vi "Listen.vi"(8 "error in (no error)":errorcluster, 11 "COGNEX IP:Port(recv)":string="192.168.0.30:4001") -> (0 "error out":errorcluster, 1 "f":string, 2 "狀態":string, 3 "Raw data":string, 4 "current time":timestamp, 5 "指示燈":bool)   [LabVIEW 2019, in "Kolmogan Library 1.lvlib"]
uses:
  Kolmogan Library 1.lvlib
  <vilib>/regexp/Match Regular Expression.xnode
panel:
  out "x-y":dbl
  out "length":i32
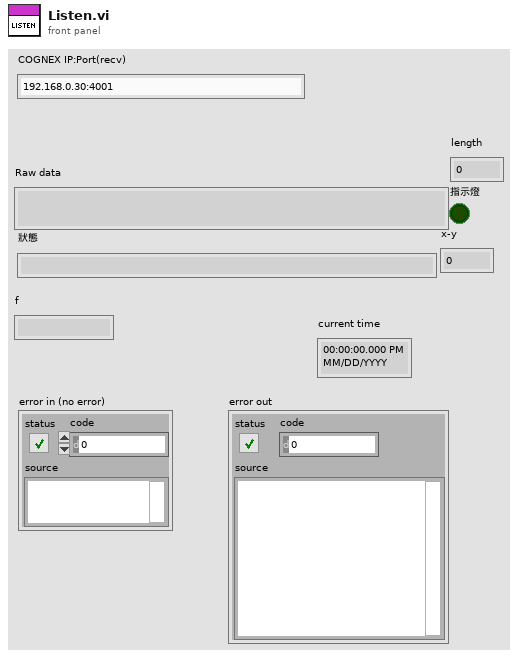
[diagram p1: front panel]
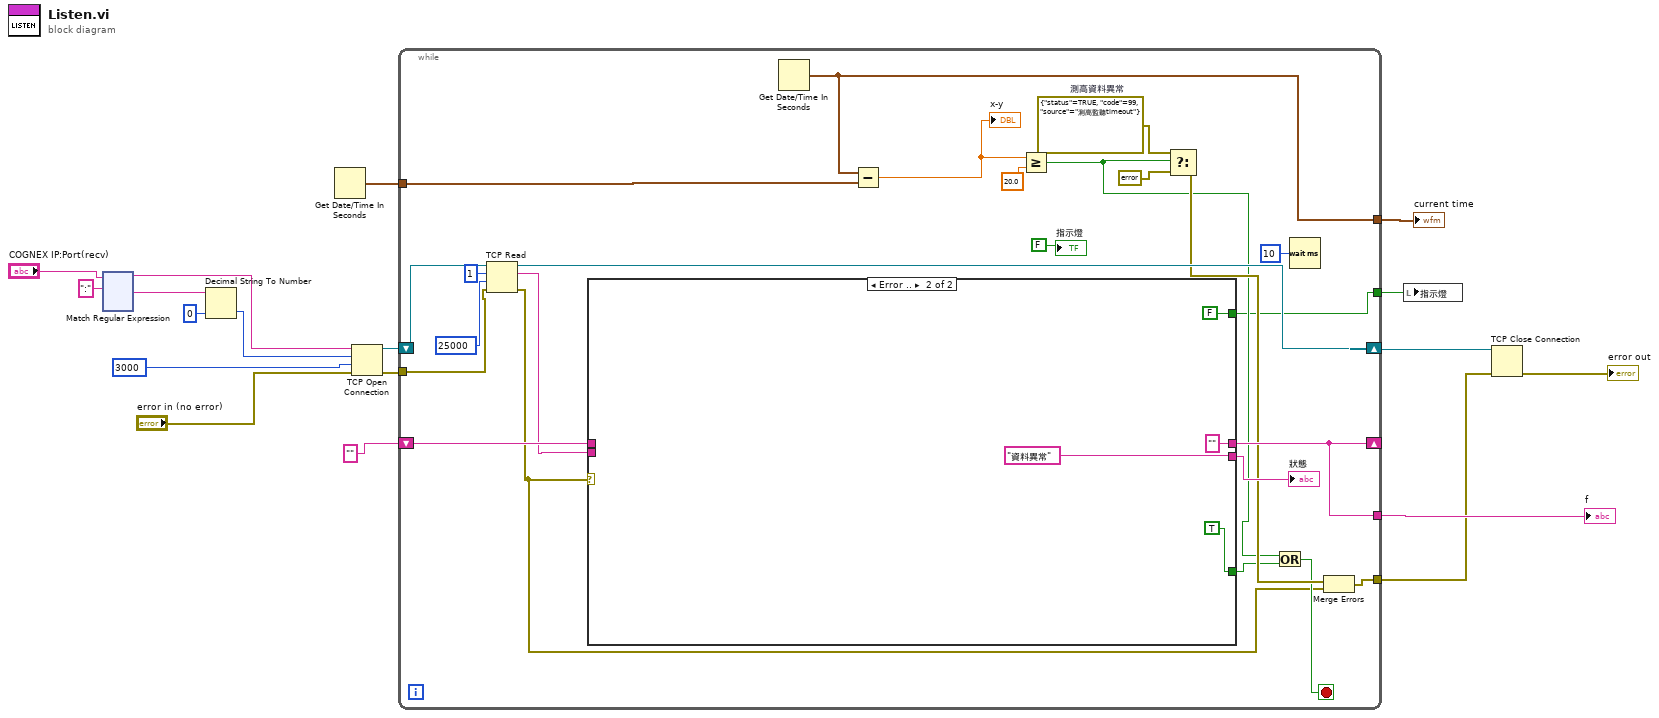
[diagram p0: block diagram]
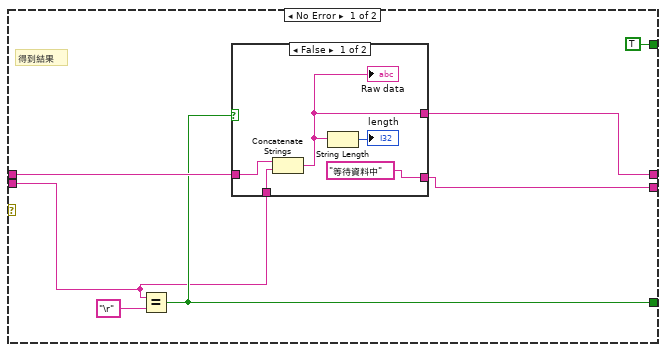
[diagram p2: hidden frame]
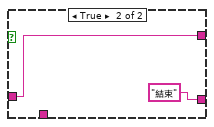
[diagram p3: hidden frame]
diagram:
  n1 = xnode "Match Regular Expression"("input string"="COGNEX IP:Port(recv)", "regular expression"=":") -> ("before match"=w3:string, "after match"=w6:string)  [unwired: 4 in, 3 out]
  n2 = Decimal String To Number(string=w6, default (0L)=u16 0 ("default (0 I32)")) -> (number=w2:u16)  [unwired: 1 in, 1 out]
  n3 = Get Date/Time In Seconds() -> (seconds since 1Jan1904=w8:timestamp)
  n4 = TCP Open Connection(address=w3, remote port or service name=w2, timeout ms (60000)=3000, error in (no error)="error in (no error)") -> (connection ID=w11:refnum<k5>, error out=w13:errorcluster)  [unwired: 1 in]
  n5 = while {
    shift-right: [w38] -> w15
    shift-left: w11 -> [w42]
    shift-right: [w32] -> _
    shift-left: "" ("string") -> [w39]
    tunnel: w13 -> [w37]
    tunnel: [w27] -> w16
    tunnel: [w32] -> w18
    tunnel: [w22] -> w10
    tunnel: [w20] -> w9
    tunnel: w8 -> [w21]
    stop <- w24 stop-if-true
    w28 = errorcluster {"status"=TRUE, "code"=99, "source"="測高監聽timeout"}  # 測高資料異常
    n6 = TCP Read(connection ID=w42, bytes to read=1, error in (no error)=w37, 9:25000 ("timeout ms (25000)")) -> (connection ID out=w38:refnum<k5>, data out=w35:string, error out=w19:errorcluster)  [unwired: 1 in]
    n7 = case shown="Error .." w19 {
      tunnel: w35 -> [w45 _]
      tunnel: w39 -> [w49 _]
      tunnel: [w48 ""] -> w32
      tunnel: [w44 "資料異常" ("f")] -> w33
      tunnel: [w46 TRUE] -> w25
      tunnel: [TRUE ("指示燈") FALSE ("指示燈")] -> w20
      frame No Error {
        # "得到結果"
        n8 = Equal?(x=w45, y="\r") -> (x = y?=w46:bool)
        n9 = case shown="False" w46 {
          tunnel: w49 -> [w54 w56]
          tunnel: [w53 w56] -> w48
          tunnel: w45 -> [w51 _]
          tunnel: ["等待資料中" ("f") "結束" ("t")] -> w44
          frame False {
            n10 = Concatenate Strings(w54, w51) -> (w53:string)
            "Raw data" <- w53
            n11 = String Length(string=w53) -> (length=→"length":i32)
          }
          frame True {
          }
        }
      }
      frame Error {
      }
    }
    "狀態" <- w33
    n12 = Get Date/Time In Seconds() -> (seconds since 1Jan1904=w22:timestamp)
    n13 = Subtract(x=w22, y=w21) -> (x-y=w31:dbl)
    "x-y" <- w31
    n14 = Greater Or Equal?(x=w31, y=20.0) -> (x >= y?=w23:bool)
    n15 = Select(t=w28, s=w23, f=errorcluster {"status"=FALSE, "code"=0, "source"=""} ("error out")) -> (s? t:f=w26:errorcluster)
    n16 = Or(x=w23, y=w25) -> (x .or. y?=w24:bool)
    n17 = Wait (ms)(milliseconds to wait=u32 10) -> ()  [unwired: 1 out]
    n18 = Merge Errors(w26, w19) -> (w27:errorcluster)
    "指示燈" <- FALSE
  }
  "f" <- w18
  "current time" <- w10
  n19 = local write "指示燈"(w9) -> ()
  n20 = TCP Close Connection(connection ID=w15, error in (no error)=w16) -> (error out=→"error out":errorcluster)  [unwired: 1 in, 1 out]
